vi "execute.vi"(8 "error in (no error)":errorcluster, 9 "data collection in":refnum<class "GenericComponent.lvclass">, 10 "imaging mode in":refnum<class "GenericComponent.lvclass">, 11 "DL090325ImagingnModeToDataCollectionAdapter in":refnum<class "AdapterDL090325ImagingModeToDataCollection.lvclass">) -> (0 "error out":errorcluster, 1 "data collection out":refnum<class "GenericComponent.lvclass">, 2 "imaging mode out":refnum<class "GenericComponent.lvclass">, 3 "DL090325ImagingModeToDataCollectionAdapter out":refnum<class "AdapterDL090325ImagingModeToDataCollection.lvclass">)   [LabVIEW 2010, in "AdapterDL090325ImagingModeToDataCollection.lvclass"]
uses:
  AdapterDL090325ImagingModeToDataCollection.lvclass
  common/classes/GenericComponent/GenericComponent/GenericComponent.lvclass
  DataCollection/DataCollectionDL090215/DataCollectionDL090215/DataCollectionDL090215.lvclass
  ImagingMode/ImagingModeDL090130Frame/ImagingModeDL090130Frame/ImagingModeDL090130Frame.lvclass
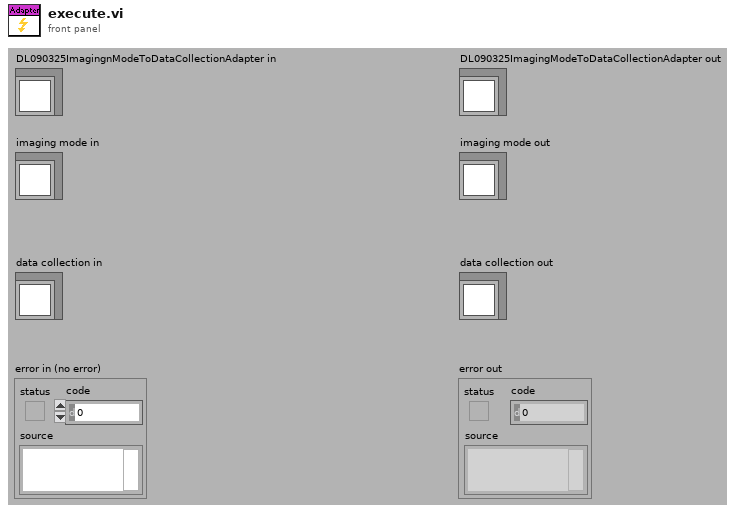
[diagram p1: front panel]
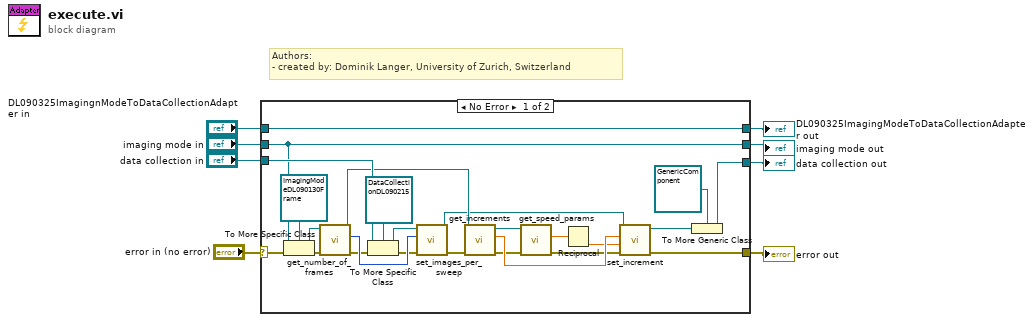
[diagram p0: block diagram]
diagram:
  # "Authors: \n- created by: Dominik Langer, University of Zurich, Switzerland"
  n1 = case shown="No Error" "error in (no error)" {
    selector: "error in (no error)" -> [w25 w37]
    tunnel: [w11 w37] -> w7
    tunnel: [w21 w36] -> w6
    tunnel: "imaging mode in" -> [w20 w34]
    tunnel: "DL090325ImagingnModeToDataCollectionAdapter in" -> [w21 w36]
    tunnel: "data collection in" -> [w24 w35]
    tunnel: [w22 w35] -> w2
    tunnel: [w20 w34] -> w1
    frame No Error {
      n2 = To More Specific Class(target class=refnum<class "ImagingModeDL090130Frame.lvclass"> refnum ("DL090130FrameScanMode.lvclass"), reference=w20, error in=w25) -> (specific class reference=w30:refnum<class "ImagingModeDL090130Frame.lvclass">, error out=w31:errorcluster)
      n3 = call-dynamic "get_number_of_frames.vi"("error in (no error)"=w31, "ImagingModeDL090130Frame in"=w30) -> ("error out"=w23:errorcluster, "number of frames"=w28:i32, "ImagingModeDL090130Frame out"=w18:refnum<class "ImagingModeDL090130Frame.lvclass">)  [unwired: 7 out]
      n4 = To More Specific Class(target class=refnum<class "DataCollectionDL090215.lvclass"> refnum ("DataCollectionDL090215.lvclass"), reference=w24, error in=w23) -> (specific class reference=w29:refnum<class "DataCollectionDL090215.lvclass">, error out=w27:errorcluster)
      n5 = call "set_images_per_sweep.vi"("error in (no error)"=w27, "images per sweep"=w28, "DataCollectionDL090215 in"=w29) -> ("error out"=w19:errorcluster, "DataCollectionDL090215 out"=w16:refnum<class "DataCollectionDL090215.lvclass">)  [unwired: 7 in]
      n6 = call-dynamic "get_increments.vi"("error in (no error)"=w19, "ImagingModeDL090130Frame in"=w18) -> ("error out"=w14:errorcluster, "step size"=w17:dbl[unit], "ImagingModeDL090130Frame out"=w15:refnum<class "ImagingModeDL090130Frame.lvclass">)  [unwired: 7 in]
      n7 = call-dynamic "get_speed_params.vi"("error in (no error)"=w14, "ImagingModeDL090130Frame in"=w15) -> ("error out"=w13:errorcluster, "frame rate"=w9:dbl[unit])  [unwired: 4 in, 4 out]
      n8 = Reciprocal(x=w9) -> (1/x=w12:dbl[unit])
      n9 = call "set_increment.vi"("error in (no error)"=w13, "time increment"=w12, "z increment"=w17, "DataCollectionDL090215 in"=w16) -> ("error out"=w11:errorcluster, "DataCollectionDL090215 out"=w10:refnum<class "DataCollectionDL090215.lvclass">)  [unwired: 6 in]
      n10 = To More Generic Class(target class=refnum<class "GenericComponent.lvclass"> refnum ("GenericComponent.lvclass"), reference=w10) -> (generic class reference=w22:refnum<class "GenericComponent.lvclass">)
    }
    frame Error {
    }
  }
  "error out" <- w7
  "DL090325ImagingModeToDataCollectionAdapter out" <- w6
  "data collection out" <- w2
  "imaging mode out" <- w1
